vi "Format TCPIP VISA Resource Name.vi"(9 "Port Number (7770)":i32=7770, 10 "Hostname or IP Address":string) -> (3 "VISA resource name out":string)   [LabVIEW 2020, in "Zaber A Series.lvlib"]
doc: "Formats a VISA resource name for use with the Initialize TCP/IP VI. \n\nUse this VI to convert a network host name or IP address and a port number into a VISA resource name string."
uses:
  Zaber A Series.lvlib
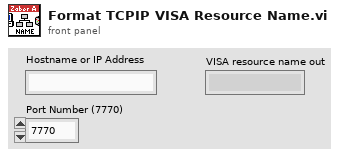
[diagram p1: front panel]
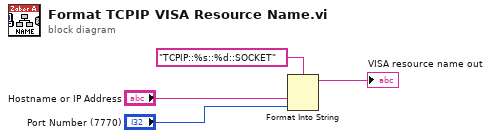
[diagram p0: block diagram]
diagram:
  n1 = Format Into String(format string="TCPIP::%s::%d::SOCKET", "Hostname or IP Address", "Port Number (7770)") -> (resulting string=→"VISA resource name out":string)  [unwired: 2 in, 1 out]
